vi "NI-DAQmx_server.vi"(5 "No of samples+extra":i32=1024 min=0 step=1) -> (15 "error out":errorcluster)   [LabVIEW 2011]
uses:
  <vilib>/DAQmx/read.llb/DAQmx Read (Analog 2D DBL NChan NSamp).vi
  Globals/Meas_global.vi
  PWA/PWAtasksGLOBAL.vi
  <vilib>/DAQmx/configure/timing.llb/DAQmx Timing (Sample Clock).vi
  <vilib>/DAQmx/create/channels.llb/DAQmx Create Channel (AI-Voltage-Basic).vi
  <vilib>/DAQmx/miscellaneous.llb/DAQmx Fill In Error Info.vi
  Program Files/National Instruments/LabVIEW 2011/resource/objmgr/daqmx.rc
panel:
  out "input terminal configuration":i32(ring)=10106 items=["default"=-1, "RSE"=10083, "NRSE"=10078, "Differential"=10106, "Pseudodifferential"=12529]
  out "AI.Voltage.Rngs":dbl[](array[numeric])=[-10.0, 10.0]
  out "TotalSampPerChanAcquired":dbl=1024.0
  out "AvailSampPerChan":u32
  out "CurrReadPos":dbl=1024.0
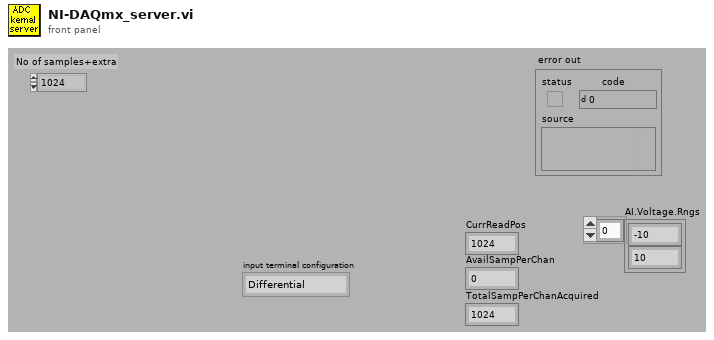
[diagram p1: front panel]
types:
  T1 = typedef "Ch_and_Spans.ctl" = cluster{"high limit (10V)":sgl, "low limit (-10V)":sgl, "Ch No":i16, "Var name":string, "Use Latest Calib":bool}
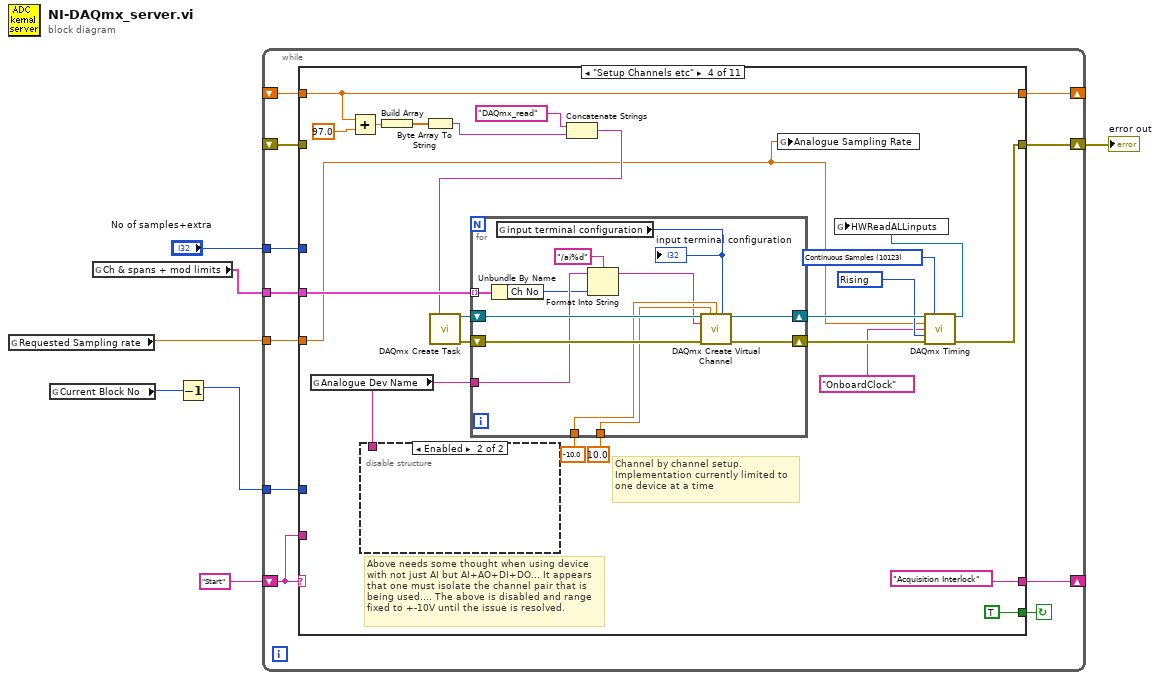
[diagram p0: block diagram]
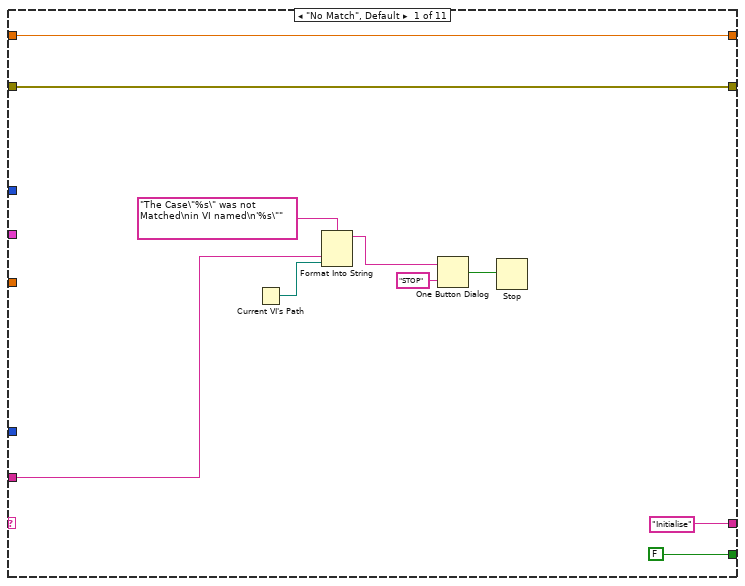
[diagram p2: hidden frame]
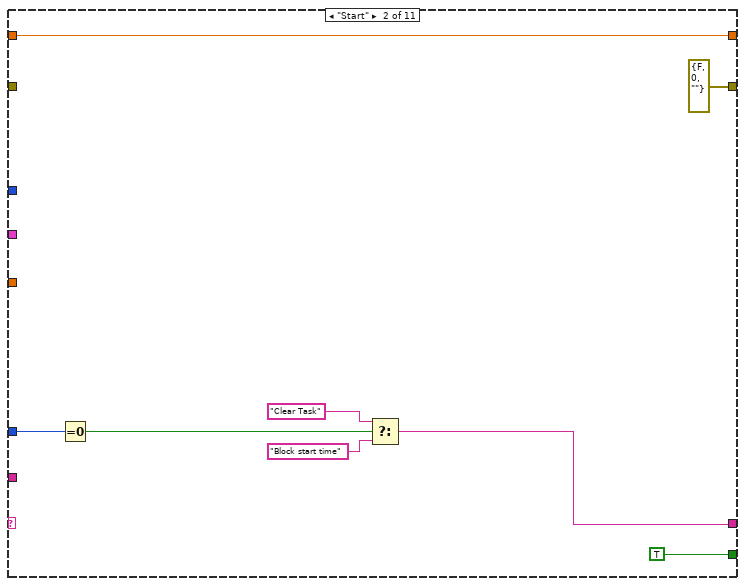
[diagram p3: hidden frame]
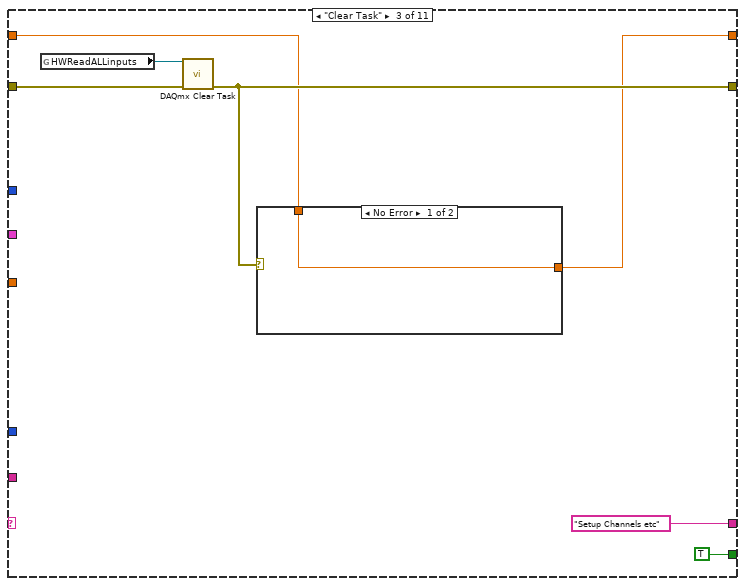
[diagram p4: hidden frame]
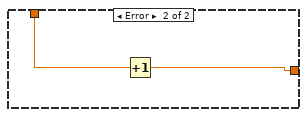
[diagram p5: hidden frame]
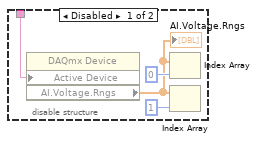
[diagram p6: hidden frame]
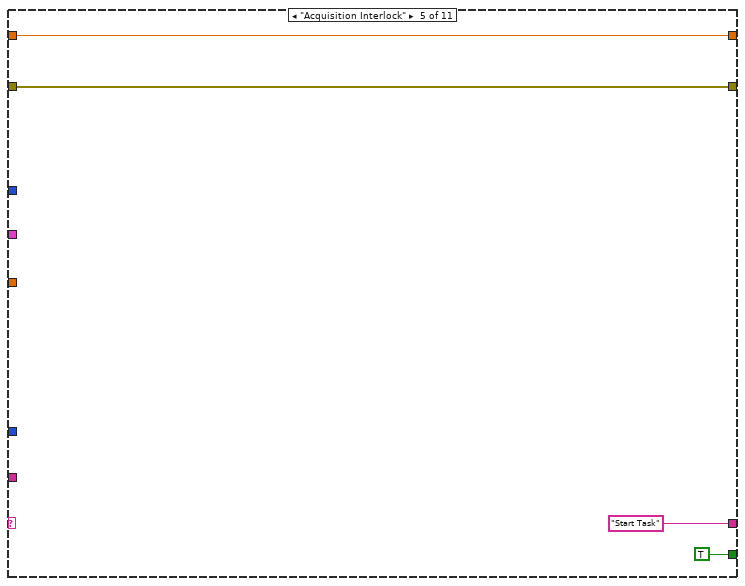
[diagram p7: hidden frame]
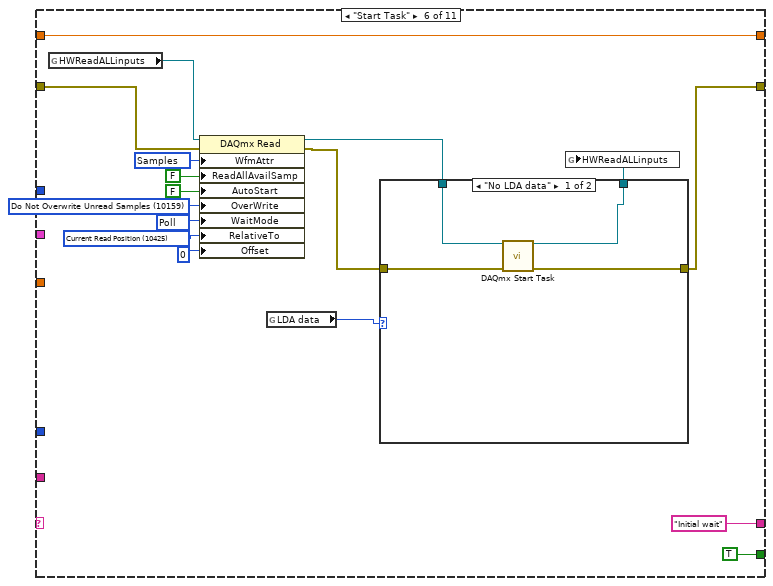
[diagram p8: hidden frame]
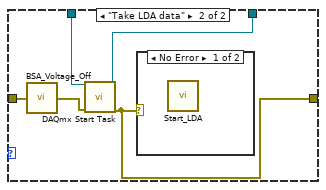
[diagram p9: hidden frame]
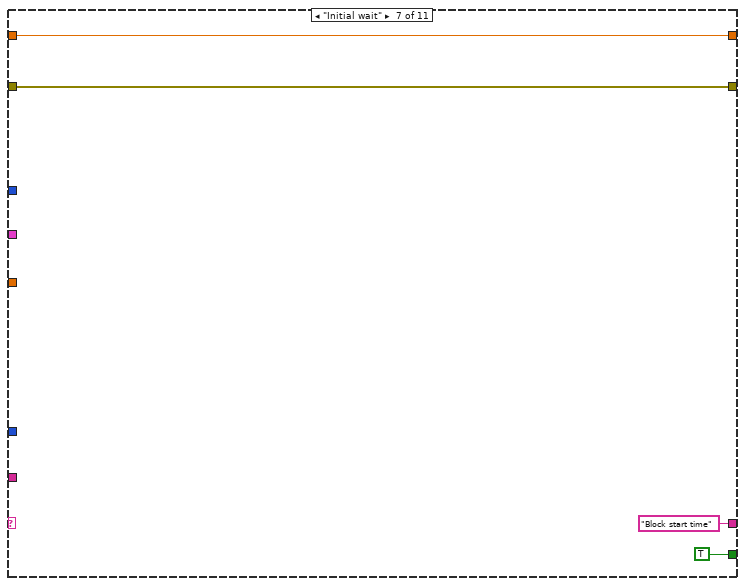
[diagram p11: hidden frame]
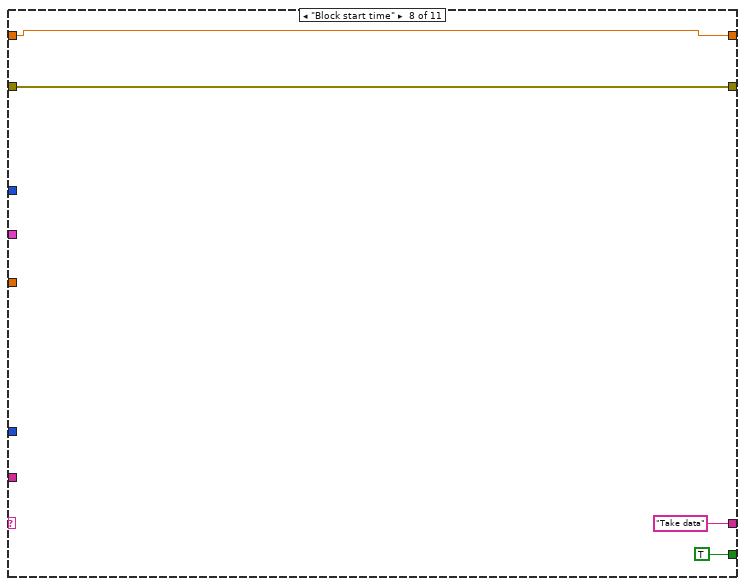
[diagram p12: hidden frame]
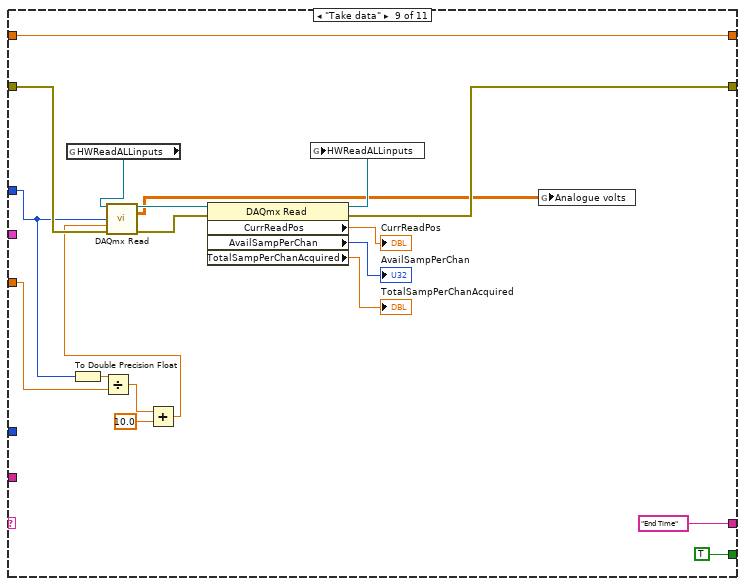
[diagram p13: hidden frame]
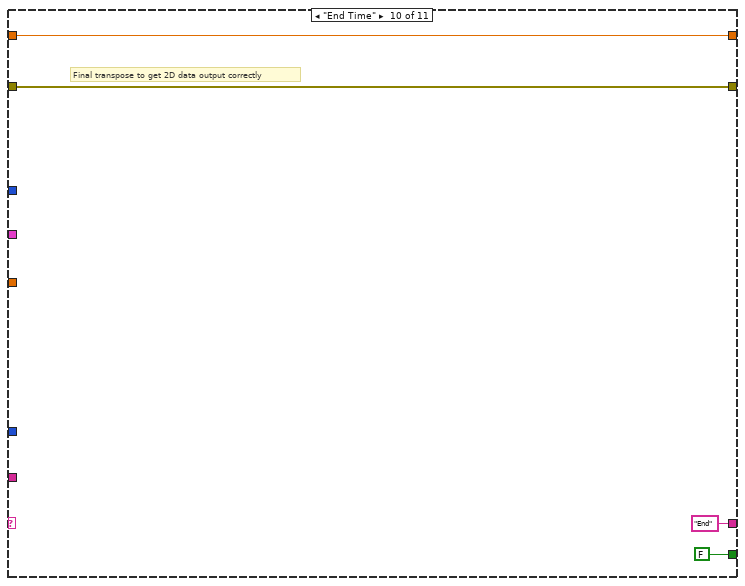
[diagram p14: hidden frame]
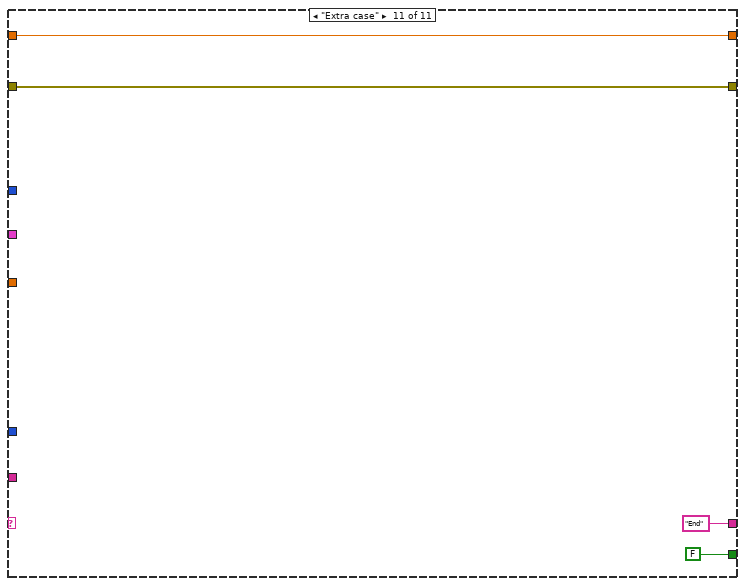
[diagram p15: hidden frame]
diagram:
  n1 = global read "Meas_global.vi" "Requested Sampling rate"() -> (w1:dbl)
  n2 = global read "Meas_global.vi" "Current Block No"() -> (w4:i32)
  n3 = global read "Meas_global.vi" "Ch & spans + mod limits"() -> (w3:T1[])
  n4 = Decrement(x=w4) -> (x-1=w2:i32)
  n5 = while {
    shift-left: "Start" -> [w16]
    shift-right: [w17] -> _
    shift-right: [w10] -> w5
    shift-left: _ -> [w15]
    tunnel: w1 -> [w14]
    tunnel: "No of samples+extra" -> [w13]
    tunnel: w2 -> [w12]
    tunnel: w3 -> [w11]
    shift-right: [w9] -> _
    shift-left: _ -> [w8]
    stop <- w18 continue-if-true
    n6 = case shown="\"Setup Channels etc\"" w16 {
      tunnel: [FALSE TRUE TRUE TRUE TRUE TRUE TRUE TRUE TRUE FALSE FALSE] -> w18
      tunnel: ["Initialise" w31 "Setup Channels etc" "Acquisition Interlock" "Start Task" "Initial wait" "Block start time" ("f") "Take data" "End Time" "End" ("f") "End" ("f")] -> w17
      tunnel: w16 -> [w23 _ _ _ _ _ _ _ _ _ _]
      tunnel: [w20 errorcluster {"status"=FALSE, "code"=0, "source"=""} ("error out") w39 w63 w88 w91 w117 w123 w136 w144 w148] -> w10
      tunnel: w15 -> [w20 _ w40 _ w88 w97 w117 w123 w142 w144 w148]
      tunnel: w14 -> [_ _ _ w47 _ _ _ _ w128 _ _]
      tunnel: w13 -> [_ _ _ _ _ _ _ _ w129 _ _]
      tunnel: w12 -> [_ w35 _ _ _ _ _ _ _ _ _]
      tunnel: w11 -> [_ _ _ w62 _ _ _ _ _ _ _]
      tunnel: [w19 w30 w38 w48 w86 w95 w116 w120 w131 w143 w147] -> w9
      tunnel: w8 -> [w19 w30 w37 w48 w86 w95 w116 w120 w131 w143 w147]
      frame "No Match", Default {
        n7 = Current VI's Path() -> (path=w22:path)
        n8 = Format Into String(format string="The Case\"%s\" was not Matched\nin VI named\n'%s\"" ("Format String"), w23, w22) -> (resulting string=w26:string)  [unwired: 2 in, 1 out]
        n9 = One Button Dialog(message=w26, button name ("OK")="STOP") -> (true=w24:bool)
        n10 = Stop(stop? (T)=w24) -> ()
      }
      frame "Start" {
        n11 = Equal To 0?(x=w35) -> (x = 0?=w32:bool)
        n12 = Select(t="Clear Task", s=w32, f="Block start time") -> (s? t:f=w31:string)
      }
      frame "Clear Task" {
        n13 = global read "PWAtasksGLOBAL.vi" "HWReadALLinputs"() -> (w41:refnum<k21>)
        n14 = call <vilib>:"DAQmx Clear Task.vi"("task in"=w41, "error in"=w40) -> ("error out"=w39:errorcluster)  [unwired: 13 out]
        n15 = case shown="No Error" w39 {
          tunnel: [w44 w45] -> w38
          tunnel: w37 -> [w44 w46]
          frame No Error {
          }
          frame Error {
            n16 = Increment(x=w46) -> (x+1=w45:dbl)
          }
        }
      }
      frame "Setup Channels etc" {
        w60 = 10280 items=["Rising"=10280, "Falling"=10171] ("active edge")
        w66 = 10123 items=["Finite Samples"=10178, "Continuous Samples"=10123, "Hardware Timed Single Point"=12522] ("sample mode")
        # "Above needs some thought when using device with not just AI but AI+AO+DI+DO... It appears that one must isolate the channel pair that is being used.... The above is disabled and range fixed to +-10V until the issue is resolved."
        # "Channel by channel setup. Implementation currently limited to one device at a time"
        n17 = global read "PWAtasksGLOBAL.vi" "Analogue Dev Name"() -> (w55:string)
        n18 = Add(x=w48, y=97.0) -> (x+y=w53:dbl)
        n19 = disable-structure shown="Enabled" {
          disable-tunnel: w55 -> [w70 _]
          frame Disabled {
            n20 = property class="DAQmx Device"("Active Device"=w70) -> ("AI.Voltage.Rngs"=w71:dbl[])  [unwired: 2 in, 2 out]
            "AI.Voltage.Rngs" <- w71
            n21 = Index Array(array=w71, index=0) -> ()  [unwired: 1 out]
            n22 = Index Array(array=w71, index=1) -> ()  [unwired: 1 out]
          }
          frame Enabled {
          }
        }
        n23 = Build Array(w53) -> (w52:dbl[])
        n24 = Byte Array To String(unsigned byte array=w52) -> (string=w50:string)
        n25 = Concatenate Strings("DAQmx_read" ("new task name"), w50) -> (w49:string)
        n26 = call <vilib>:"DAQmx Create Task.vi"("new task name"=w49) -> ("task out"=w64:refnum<k21>, "error out"=w67:errorcluster)  [unwired: 4 in, 9 out]
        n27 = for {
          tunnel: w62 -> [w85] mode=indexing
          shift-right: [w83] -> w65
          shift-left: w64 -> [w84]
          shift-right: [w81] -> w68
          shift-left: w67 -> [w82]
          tunnel: w55 -> [w78]
          tunnel: -10.0 -> [w80]
          tunnel: 10.0 -> [w79]
          n28 = Unbundle By Name(w85) -> ("Ch No"=w77:i16)
          n29 = global read "Meas_global.vi" "input terminal configuration"() -> (w74:i32)
          "input terminal configuration" <- w74
          n30 = Format Into String(format string="/ai%d", initial string=w78, w77) -> (resulting string=w75:string)  [unwired: 1 in, 1 out]
          n31 = call-poly <vilib>:"DAQmx Create Virtual Channel.vi"("task in"=w84, "maximum value"=w79, "minimum value"=w80, "input terminal configuration"=w74, "physical channels"=w75, "error in"=w82) -> ("task out"=w83:refnum<k21>, "error out"=w81:errorcluster)  [unwired: 3 in, 5 out]
        }
        n32 = global write "Meas_global.vi" "Analogue Sampling Rate"(w47) -> ()
        n33 = call-poly <vilib>:"DAQmx Timing.vi"("task/channels in"=w65, "sample mode"=w66, "rate"=w47, "source"=tag "OnboardClock", "active edge"=w60, "error in"=w68) -> ("task out"=w61:refnum<k21>, "error out"=w63:errorcluster)  [unwired: 1 in, 7 out]
        n34 = global write "PWAtasksGLOBAL.vi" "HWReadALLinputs"(w61) -> ()
      }
      frame "Acquisition Interlock" {
      }
      frame "Start Task" {
        w100 = 10425 items=["First Sample"=10424, "Current Read Position"=10425, "Reference Trigger"=10426, "First Pretrigger Sample"=10427, "Most Recent Sample"=10428] ("RelativeTo")
        w101 = 12524 items=["Wait For Interrupt"=12523, "Poll"=12524, "Yield"=12525, "Sleep"=12547] ("WaitMode")
        w102 = 10159 items=["Overwrite Unread Samples"=10252, "Do Not Overwrite Unread Samples"=10159] ("OverWrite")
        w104 = 10287 items=["Samples"=10287, "Samples and Timing"=10140, "Samples, Timing, and Attributes"=10141] ("WfmAttr")
        n35 = global read "PWAtasksGLOBAL.vi" "HWReadALLinputs"() -> (w98:refnum<k21>)
        n36 = property class="DAQmx Read"(reference=w98, error in=w97, "WfmAttr"=w104, "ReadAllAvailSamp"=FALSE, "AutoStart"=FALSE, "OverWrite"=w102, "WaitMode"=w101, "RelativeTo"=w100, "Offset"=0) -> (reference out=w92:refnum<k21>, error out=w93:errorcluster)
        n37 = global read "Meas_global.vi" "LDA data"() -> (w94:enum16{"No LDA data", "Take LDA data"})
        n38 = case shown="\"No LDA data\"" w94 {
          tunnel: w93 -> [w110 w115]
          tunnel: [w107 w112] -> w91
          tunnel: w92 -> [w109 w113]
          tunnel: [w108 w111] -> w90
          frame "No LDA data" {
            n39 = call <vilib>:"DAQmx Start Task.vi"("task/channels in"=w109, "error in"=w110) -> ("task out"=w108:refnum<k21>, "error out"=w107:errorcluster)  [unwired: 12 out]
          }
          frame "Take LDA data" {
            n40 = call "BSA_Voltage_Off.vi"("error in"=w115) -> ("error out"=w114:errorcluster)
            n41 = call <vilib>:"DAQmx Start Task.vi"("task/channels in"=w113, "error in"=w114) -> ("task out"=w111:refnum<k21>, "error out"=w112:errorcluster)  [unwired: 12 out]
            n42 = case shown="No Error" w112 {
              frame No Error {
                n43 = call "Start_LDA.vi"() -> ()  [unwired: 1 out]
              }
              frame Error {
              }
            }
          }
        }
        n44 = global write "PWAtasksGLOBAL.vi" "HWReadALLinputs"(w90) -> ()
      }
      frame "Initial wait" {
      }
      frame "Block start time" {
      }
      frame "Take data" {
        n45 = global read "PWAtasksGLOBAL.vi" "HWReadALLinputs"() -> (w134:refnum<k21>)
        n46 = To Double Precision Float(number=w129) -> (double precision float=w130:dbl)
        n47 = Divide(x=w130, y=w128) -> (x/y=w127:dbl)
        n48 = Add(x=w127, y=10.0) -> (x+y=w125:dbl)
        n49 = call-poly <vilib>:"DAQmx Read.vi"("task/channels in"=w134, "number of samples per channel"=w129, "timeout"=w125, "error in"=w142) -> ("task out"=w139:refnum<k21>, "data"=w124:dbl[][], "error out"=w133:errorcluster)  [unwired: 9 out]
        n50 = property class="DAQmx Read"(reference=w139, error in=w133) -> (reference out=w138:refnum<k21>, error out=w136:errorcluster, "CurrReadPos"=→"CurrReadPos":dbl, "AvailSampPerChan"=→"AvailSampPerChan":u32, "TotalSampPerChanAcquired"=→"TotalSampPerChanAcquired":dbl)
        n51 = global write "PWAtasksGLOBAL.vi" "HWReadALLinputs"(w138) -> ()
        n52 = global write "Meas_global.vi" "Analogue volts"(w124) -> ()
      }
      frame "End Time" {
        # "Final transpose to get 2D data output correctly"
      }
      frame "Extra case" {
      }
    }
  }
  "error out" <- w5
